vi "DAY 5 Mini UI to Replicate Real System.vi"() -> ()   [LabVIEW 2026]
panel:
  out "Fuel Reserve %":u8(slide) scale=0.0..100.0
  out "Current Engine RPM":dbl(knob) scale=0.0..10.0
  in  "Target Velocity (Mach)":dbl(slide) scale=0.0..10.0
  # "SYSTEMS & PROPULSION TELEMETRY"
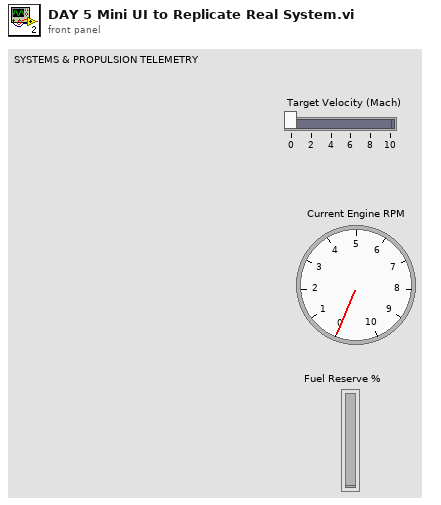
[diagram p1: front panel]
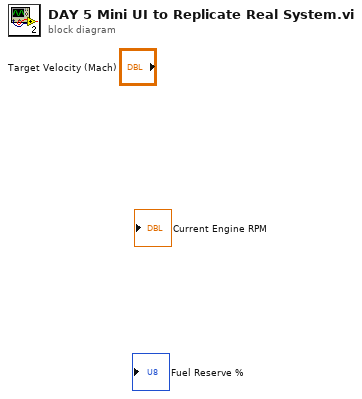
[diagram p0: block diagram]
diagram:
